vi "WriteToSpreadsheetFile(DBL)[MM].vi"(4 "transpose? (no:F)":bool, 5 "format (%.3f)":string="%.3f", 6 "append to file? (new file:F)":bool, 7 "delimiter (\\t)":string="\t", 8 "error in":errorcluster, 9 "1D data":dbl[](array[numeric]) format="%0.2f", 10 "2D data":dbl[][](array[numeric]) format="%0.2f", 11 "file path (dialog if empty)":path) -> (0 "error out":errorcluster, 2 "Done":bool, 3 "new file path (Not A Path if cancelled)":path)   [LabVIEW 2013]
doc: "Converts a 2D or 1D array of strings, signed integers, or double-precision numbers to a text string and writes the string to a new byte stream file or appends the string to an existing file. Wire data to the <B>2D data</B> input or <B>1D data</B> input to determine the polymorphic instance to use or manually select the instance.\n\nUse this VI to transpose or separate data.\n\n<B>Note</B> This is a modified version with the error handling enabled"
panel:
  in  "prompt":string="Choose file to write."
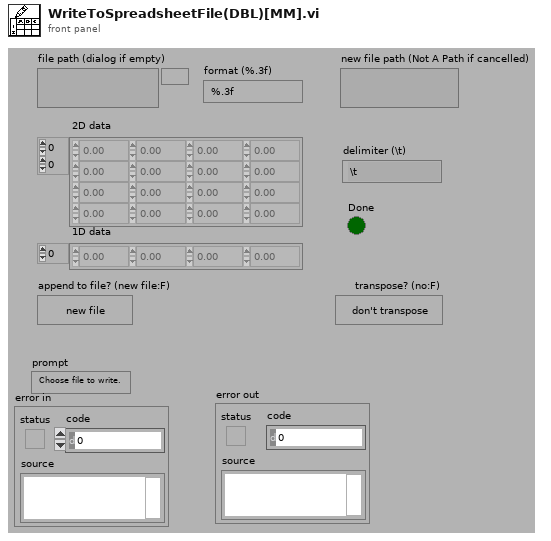
[diagram p1: front panel]
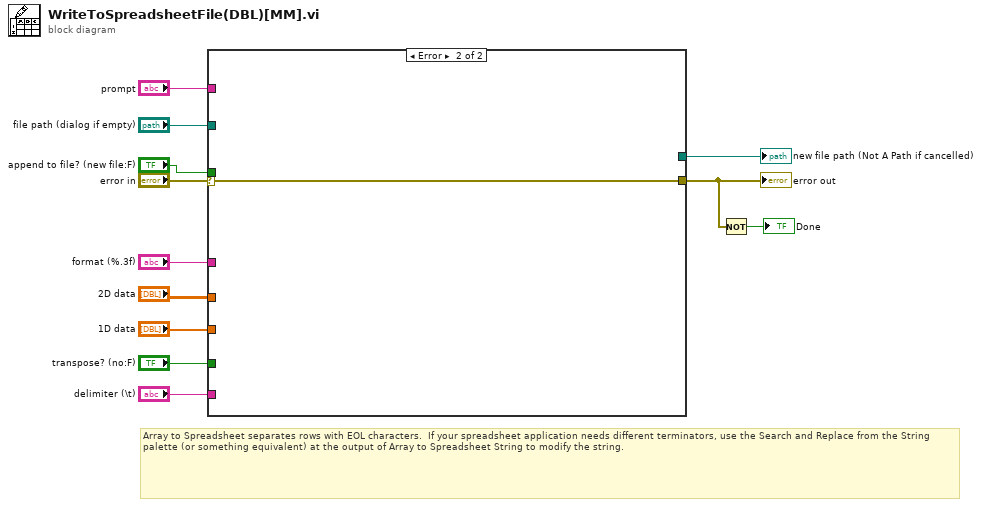
[diagram p0: block diagram]
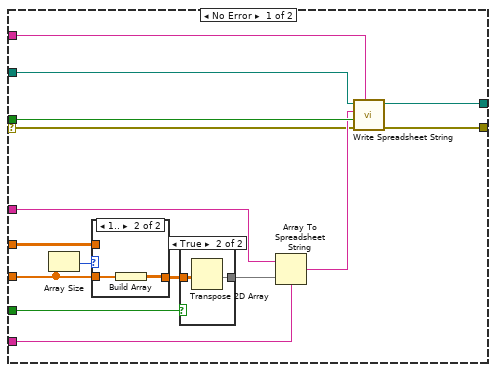
[diagram p2: hidden frame]
diagram:
  # "Array to Spreadsheet separates rows with EOL characters.  If your spreadsheet application needs different terminators, use the Search and Replace from the String palette (or something equivalent) at the output of Array to Spreadsheet String to modify the string."
  n1 = case shown="Error" "error in" {
    selector: "error in" -> [w13 w34]
    tunnel: "append to file? (new file:F)" -> [w27 _]
    tunnel: "1D data" -> [w25 _]
    tunnel: "2D data" -> [w24 _]
    tunnel: "format (%.3f)" -> [w23 _]
    tunnel: "transpose? (no:F)" -> [w21 _]
    tunnel: "file path (dialog if empty)" -> [w19 _]
    tunnel: "delimiter (\\t)" -> [w18 _]
    tunnel: "prompt" -> [w17 _]
    tunnel: [w16 _] -> w4
    tunnel: [w14 w34] -> w2
    frame No Error {
      n2 = Array Size(array=w25) -> (size(s)=w26:i32)
      n3 = case shown="1.." w26 {
        tunnel: w25 -> [_ w33]
        tunnel: [w31 w32] -> w22
        tunnel: w24 -> [w31 _]
        frame ..0 {
          # "1D array is empty"
        }
        frame 1.. {
          n4 = Build Array(w33) -> (w32:dbl[][])
        }
      }
      n5 = case shown="True" w21 {
        tunnel: [w28 w30] -> w20
        tunnel: w22 -> [w28 w29]
        frame False {
        }
        frame True {
          n6 = Transpose 2D Array(2D array=w29) -> (transposed array=w30:dbl[][])
        }
      }
      n7 = Array To Spreadsheet String(delimiter (Tab)=w18, array=w20, 3:w23) -> (spreadsheet string=w15:string)
      n8 = call "Write Spreadsheet String.vi"("prompt"=w17, "error in"=w13, "append to file? (new file:F)"=w27, "spreadsheet string"=w15, "file path (dialog if empty)"=w19) -> ("error out"=w14:errorcluster, "path"=w16:path)  [unwired: 5 in]
    }
    frame Error {
    }
  }
  "new file path (Not A Path if cancelled)" <- w4
  "error out" <- w2
  n9 = Not(x=w2) -> (.not. x?=→"Done":bool)
